vi "TIFF-Initialize Stack.vi"(0 "height":u32, 5 "width":u32, 9 "[IN] byte order":T2(ring)=enum."little-endian", 11 "error in":errorcluster) -> (4 "state":T1={"file"=refnum, "IFD"=[], "offset"=0, "byte order"=enum."little-endian", "image size"=0, "IFD size"=0, "max frames"=0, "frames"=0}, 15 "error out":errorcluster)   [LabVIEW 2020]
uses:
  TIFF-Write State.ctl
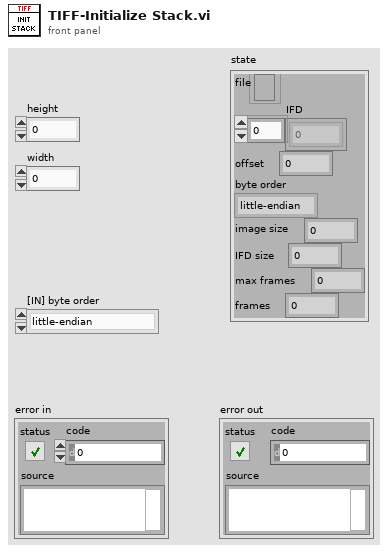
[diagram p1: front panel]
types:
  T1 = typedef "TIFF-Write State.ctl" = cluster{"file":refnum<file>, "IFD":u8[], "offset":u32, "byte order":enum16{"big-endian, network order", "native, host order", "little-endian"}, "image size":u32, "IFD size":u32, "max frames":u32, "frames":u32}
  T2 = enum16{"big-endian, network order", "native, host order", "little-endian"}
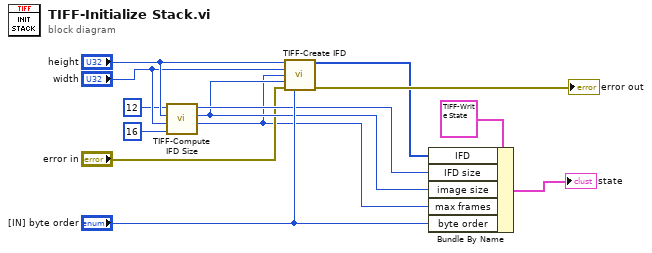
[diagram p0: block diagram]
diagram:
  n1 = call "TIFF-Compute IFD Size.vi"("[IN] Bits per sample"=u32 16, "[IN] Image width"="width", "[IN] Image length"="height", "[IN] Tags in IFD"=u32 12) -> ("max frames"=w1:u32, "[OUT] Image size in bytes"=w4:u32, "[OUT] IFD size in bytes"=w5:u32)  [unwired: 5 in]
  n2 = call "TIFF-Create IFD.vi"("height"="height", "width"="width", "max frames"=w1, "Image size (bytes)"=w4, "error in"="error in", "byte order"="[IN] byte order") -> ("unsigned byte array"=w11:u8[], "error out"=→"error out":errorcluster)  [unwired: 8 in]
  n3 = Bundle By Name(cluster=T1 {"file"=refnum, "IFD"=[], "offset"=0, "byte order"=enum."little-endian", "image size"=0, "IFD size"=0, "max frames"=0, "frames"=0} ("state"), "IFD"=w11, "IFD size"=w5, "image size"=w4, "max frames"=w1, "byte order"="[IN] byte order") -> (→"state":T1)
